vi "Get Json Status.vi"(11 "logger":cluster{"time":string, "message":string}[](array[cluster])) -> (3 "out":string)   [LabVIEW 2019]
uses:
  RT Controls/FPGA State.ctl
  RT Controls/Main Box Config.ctl
  RT Controls/Main Box Status.ctl
  RT Controls/Rotation Status.ctl
  RT Controls/Last Rotation.ctl
  RT Controls/Homing State.ctl
panel:
  out "mainHostAddr":string
  out "logs":cluster{"time":string[], "messages":string[]}
  out "messages":string[](array[string])
  out "time":string[](array[string])
  out "AZEncCounts":u64
  out "watchdogTime":bool
  out "shutdown":bool
  out "current time":timestamp
  out "antWifi":bool
  out "hostComms":bool
  out "buttons":T1
  out "config":T2
  out "errors":T3
  out "time":string
  out "AZPosError":dbl
  out "AZPosReq":dbl
  out "homed":bool
  out "homing":bool
  out "cmd":i8
  out "homeSensor":bool
  out "envSensor":bool
  out "AZEncStatus":u16
  out "subMode":u8
  out "mode":string
  out "modeReq":string
  out "AZLastRot":string
  out "AZPos":dbl
  out "AZEncCounts":u64
  out "autoShutEn":bool
  out "watchdogTim":i32
  out "topBoxComms":bool
  out "hostTimeout":bool
  out "topBoxTimeout":bool
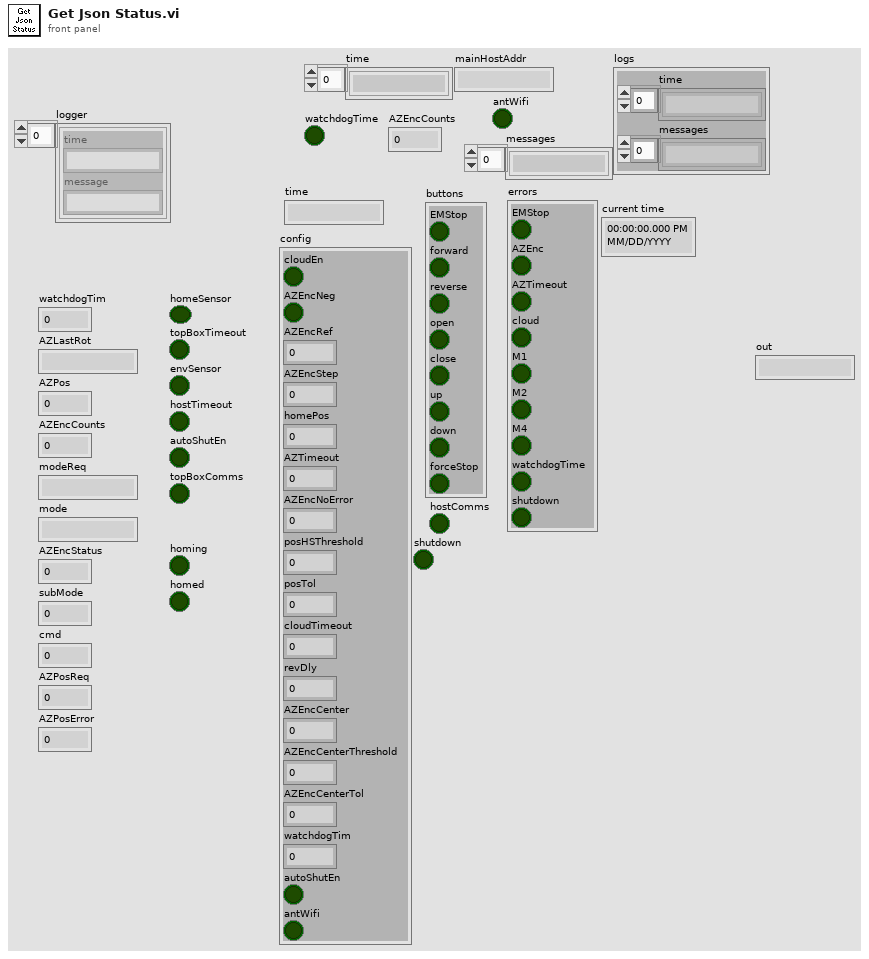
[diagram p1: front panel]
types:
  T1 = cluster{"EMStop":bool, "forward":bool, "reverse":bool, "open":bool, "close":bool, "up":bool, "down":bool, "forceStop":bool}
  T2 = cluster{"cloudEn":bool, "AZEncNeg":bool, "AZEncRef":u64, "AZEncStep":u64, "homePos":dbl, "AZTimeout":u32, "AZEncNoError":u16, "posHSThreshold":dbl, "posTol":dbl, "cloudTimeout":u32, "revDly":u32, "AZEncCenter":u64, "AZEncCenterThreshold":u64, "AZEncCenterTol":u64, "watchdogTim":i32, "autoShutEn":bool, "antWifi":bool}
  T3 = cluster{"EMStop":bool, "AZEnc":bool, "AZTimeout":bool, "cloud":bool, "M1":bool, "M2":bool, "M4":bool, "watchdogTime":bool, "shutdown":bool}
  T4 = typedef "Main Box Status.ctl" = cluster{"RotStatus":T5, "EMButton":bool, "TopComms":bool, "CurAZ":dbl, "At Home":bool, "LastRot":T6, "Cloud":bool, "CurAZEnc":u64, "LastAZ":dbl, "AutoShut":bool, "WDTime":bool, "HomeState":T7}
  T5 = typedef "Rotation Status.ctl" = enum16{"Stop", "Left", "Right", "Homing"}
  T6 = typedef "Last Rotation.ctl" = enum16{"--", "RR", "RL"}
  T7 = typedef "Homing State.ctl" = enum16{"Idle", "SlewFwd", "SlewRev", "SeekFwd", "SeekRev", "AtHome", "FwdWait", "RevWait"}
  T8 = typedef "Main Box Config.ctl" = cluster{"WatchdogTim":i32, "DirRevDel":i32, "Coast":dbl, "HSThres":dbl, "EncCounts360":u64, "HomePos":dbl, "EncRefDeg":dbl, "EncRefCounts":u64, "Tol":dbl, "CloudEn":bool, "AutoShutEn":bool, "RainTim":i32, "AZTimeout":i32, "AZEncPol":enum16{"Positive", "Negative"}}
  T9 = typedef "FPGA State.ctl" = cluster{"mode request":enum16{"stop", "home", "position", "center"}, "az last rotation":enum16{"none", "forward", "reverse"}, "emergency stop":bool, "error?":bool, "errors":cluster{"emergency stop":bool, "encoder":bool, "az timeout":bool, "m1":bool, "m2":bool, "m4":bool}, "az enc counts":u64, "az pos":fxp<+/-,32,2>, "mode":u8, "sub mode":u8, "enc status":u16, "buttons":cluster{"em-stop":bool, "forward":bool, "reverse":bool, "open":bool, "close":bool, "up":bool, "down":bool, "force stop":bool}, "cloud?":bool, "cloud to counter":u32, "az to counter":u32, "env sensor":bool, "home sensor":bool, "rev dly counter":u32, "cmd request":i8, "cmd":i8, "config":cluster{"io.cloud-enable":bool, "io.encoder-negate":bool, "io.encoder-ref":u64, "io.encoder-step":u64, "io.home-pos":fxp<+/-,32,2>, "sm.az-timeout (ms)":u32, "sm.encoder-no-error":u16, "sm.main-pos-hs-thres":fxp<+/-,32,2>, "sm.main-pos-tol":fxp<+/-,32,2>, "sm.cloud-timeout (ms)":u32, "sm.rev-dly (ms)":u32, "io.encoder-center":u64, "sm-main-center-hs-thres":u64, "sm-main-center-tol":u64}, "homing?":bool, "homed?":bool, "az pos req":fxp<+/-,32,2>, "homing wait counter":u32, "config out":cluster{"io.cloud-enable":bool, "io.encoder-negate":bool, "io.encoder-ref":u64, "io.encoder-step":u64, "io.home-pos":fxp<+/-,32,2>, "sm.az-timeout (ms)":u32, "sm.encoder-no-error":u16, "sm.main-pos-hs-thres":fxp<+/-,32,2>, "sm.main-pos-tol":fxp<+/-,32,2>, "sm.cloud-timeout (ms)":u32, "sm.rev-dly (ms)":u32, "io.encoder-center":u64, "sm-main-center-hs-thres":u64, "sm-main-center-tol":u64}, "Chassis Temperature":i16}
  T10 = cluster{"emergency stop":bool, "encoder":bool, "az timeout":bool, "m1":bool, "m2":bool, "m4":bool}
  T11 = cluster{"io.cloud-enable":bool, "io.encoder-negate":bool, "io.encoder-ref":u64, "io.encoder-step":u64, "io.home-pos":fxp<+/-,32,2>, "sm.az-timeout (ms)":u32, "sm.encoder-no-error":u16, "sm.main-pos-hs-thres":fxp<+/-,32,2>, "sm.main-pos-tol":fxp<+/-,32,2>, "sm.cloud-timeout (ms)":u32, "sm.rev-dly (ms)":u32, "io.encoder-center":u64, "sm-main-center-hs-thres":u64, "sm-main-center-tol":u64}
  T12 = cluster{"em-stop":bool, "forward":bool, "reverse":bool, "open":bool, "close":bool, "up":bool, "down":bool, "force stop":bool}
  T13 = cluster{"time":string, "hostComms":bool, "topBoxComms":bool, "mainHostAddr":string, "AZPos":dbl, "AZPosReq":dbl, "AZPosError":dbl, "AZEncCounts":u64, "AZEncStatus":u16, "AZLastRot":string, "mode":string, "modeReq":string, "subMode":u8, "cmd":i8, "buttons":cluster{"EMStop":bool, "forward":bool, "reverse":bool, "open":bool, "close":bool, "up":bool, "down":bool, "forceStop":bool}, "envSensor":bool, "homed":bool, "homing":bool, "homeSensor":bool, "config":cluster{"cloudEn":bool, "AZEncNeg":bool, "AZEncRef":u64, "AZEncStep":u64, "homePos":dbl, "AZTimeout":u32, "AZEncNoError":u16, "posHSThreshold":dbl, "posTol":dbl, "cloudTimeout":u32, "revDly":u32, "AZEncCenter":u64, "AZEncCenterThreshold":u64, "AZEncCenterTol":u64, "watchdogTim":i32, "autoShutEn":bool, "antWifi":bool}, "errors":cluster{"EMStop":bool, "AZEnc":bool, "AZTimeout":bool, "cloud":bool, "M1":bool, "M2":bool, "M4":bool, "watchdogTime":bool, "shutdown":bool}, "logs":cluster{"time":string[], "messages":string[]}}
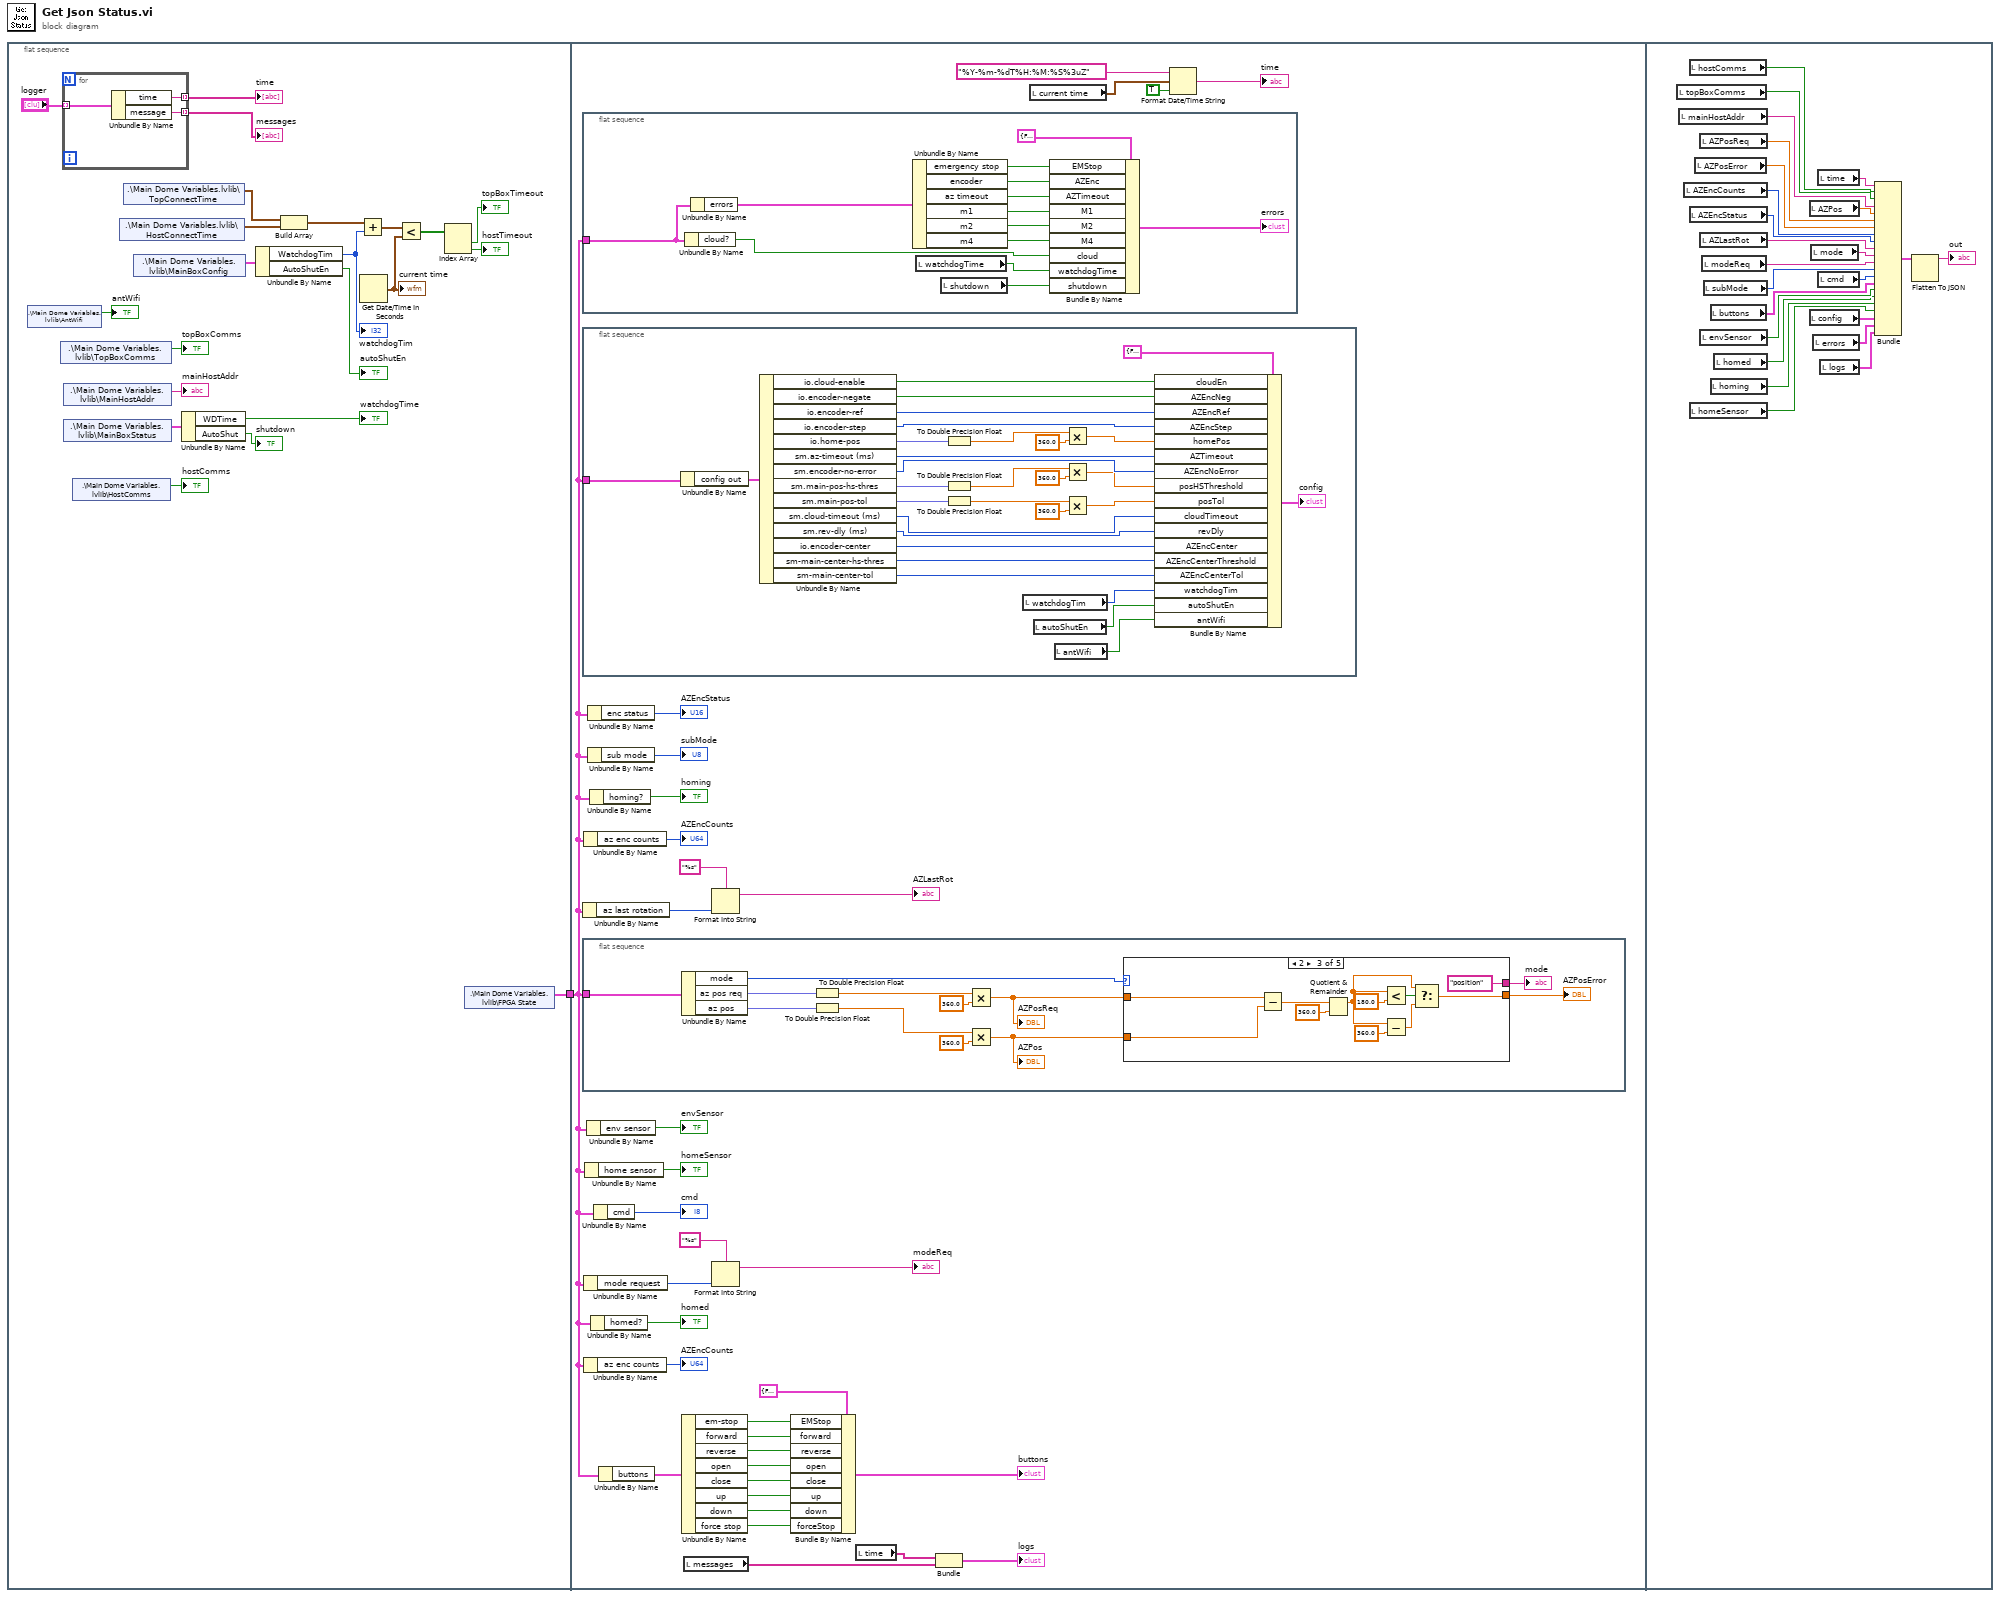
[diagram p0: block diagram]
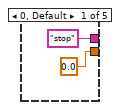
[diagram p2: hidden frame]
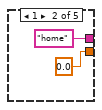
[diagram p3: hidden frame]
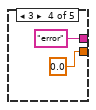
[diagram p4: hidden frame]
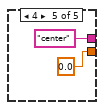
[diagram p5: hidden frame]
diagram:
  n1 = flat-sequence {
    tunnel: [w12] -> w1
    tunnel: w1 -> [w31]
    frame #0 {
      n2 = shared-variable ".\\Main Dome Variables.lvlib\\AntWifi"() -> (→"antWifi":bool)  [unwired: 1 in, 1 out]
      n3 = shared-variable ".\\Main Dome Variables.lvlib\\TopBoxComms"() -> (→"topBoxComms":bool)  [unwired: 1 in, 1 out]
      n4 = for {
        tunnel: "logger" -> [w26] mode=indexing
        tunnel: [w25] -> w4 mode=indexing
        tunnel: [w24] -> w3 mode=indexing
        n5 = Unbundle By Name(w26) -> ("time"=w25:string, "message"=w24:string)
      }
      "time" <- w4
      "messages" <- w3
      n6 = shared-variable ".\\Main Dome Variables.lvlib\\MainHostAddr"() -> (→"mainHostAddr":string)  [unwired: 1 in, 1 out]
      n7 = shared-variable ".\\Main Dome Variables.lvlib\\MainBoxStatus"() -> (w8:T4)  [unwired: 1 in, 1 out]
      n8 = shared-variable ".\\Main Dome Variables.lvlib\\HostComms"() -> (→"hostComms":bool)  [unwired: 1 in, 1 out]
      n9 = shared-variable ".\\Main Dome Variables.lvlib\\HostConnectTime"() -> (w19:timestamp)  [unwired: 1 in, 1 out]
      n10 = shared-variable ".\\Main Dome Variables.lvlib\\TopConnectTime"() -> (w20:timestamp)  [unwired: 1 in, 1 out]
      n11 = shared-variable ".\\Main Dome Variables.lvlib\\MainBoxConfig"() -> (w18:T8)  [unwired: 1 in, 1 out]
      n12 = Unbundle By Name(w8) -> ("WDTime"=→"watchdogTime":bool, "AutoShut"=→"shutdown":bool)
      n13 = Unbundle By Name(w18) -> ("WatchdogTim"=w22:i32, "AutoShutEn"=→"autoShutEn":bool)
      "watchdogTim" <- w22
      n14 = Build Array(w20, w19) -> (w21:timestamp[])
      n15 = Add(x=w21, y=w22) -> (x+y=w23:timestamp[])
      n16 = Get Date/Time In Seconds() -> (seconds since 1Jan1904=w11:timestamp)
      "current time" <- w11
      n17 = Less?(x=w23, y=w11) -> (x < y?=w17:bool[])
      n18 = Index Array(array=w17) -> (element #1=→"topBoxTimeout":bool, element #2=→"hostTimeout":bool)  [unwired: 2 in]
      n19 = shared-variable ".\\Main Dome Variables.lvlib\\FPGA State"() -> (w12:T9)  [unwired: 1 in, 1 out]
    }
    frame #1 {
      n20 = flat-sequence {
        tunnel: w31 -> [w126]
        frame #0 {
          n21 = Unbundle By Name(w126) -> ("cloud?"=w125:bool)
          n22 = Unbundle By Name(w126) -> ("errors"=w134:T10)
          n23 = Unbundle By Name(w134) -> ("emergency stop"=w132:bool, "encoder"=w131:bool, "az timeout"=w130:bool, "m1"=w129:bool, "m2"=w128:bool, "m4"=w127:bool)
          n24 = local read "watchdogTime"() -> (w122:bool)
          n25 = local read "shutdown"() -> (w123:bool)
          n26 = Bundle By Name(cluster=T3 {"EMStop"=FALSE, "AZEnc"=FALSE, "AZTimeout"=FALSE, "cloud"=FALSE, "M1"=FALSE, "M2"=FALSE, "M4"=FALSE, "watchdogTime"=FALSE, "shutdown"=FALSE} ("errors"), "EMStop"=w132, "AZEnc"=w131, "AZTimeout"=w130, "M1"=w129, "M2"=w128, "M4"=w127, "cloud"=w125, "watchdogTime"=w122, "shutdown"=w123) -> (→"errors":T3)
        }
      }
      n27 = flat-sequence {
        tunnel: w31 -> [w95]
        frame #0 {
          n28 = Unbundle By Name(w95) -> ("config out"=w121:T11)
          n29 = Unbundle By Name(w121) -> ("io.cloud-enable"=w119:bool, "io.encoder-negate"=w118:bool, "io.encoder-ref"=w117:u64, "io.encoder-step"=w116:u64, "io.home-pos"=w105:fxp<+/-,32,2>, "sm.az-timeout (ms)"=w115:u32, "sm.encoder-no-error"=w114:u16, "sm.main-pos-hs-thres"=w103:fxp<+/-,32,2>, "sm.main-pos-tol"=w101:fxp<+/-,32,2>, "sm.cloud-timeout (ms)"=w113:u32, "sm.rev-dly (ms)"=w112:u32, "io.encoder-center"=w111:u64, "sm-main-center-hs-thres"=w110:u64, "sm-main-center-tol"=w109:u64)
          n30 = To Double Precision Float(number=w105) -> (double precision float=w98:dbl)
          n31 = To Double Precision Float(number=w103) -> (double precision float=w97:dbl)
          n32 = To Double Precision Float(number=w101) -> (double precision float=w96:dbl)
          n33 = local read "watchdogTim"() -> (w108:i32)
          n34 = local read "autoShutEn"() -> (w94:bool)
          n35 = local read "antWifi"() -> (w92:bool)
          n36 = Multiply(x=w98, y=360.0) -> (x*y=w106:dbl)
          n37 = Multiply(x=w97, y=360.0) -> (x*y=w100:dbl)
          n38 = Multiply(x=w96, y=360.0) -> (x*y=w99:dbl)
          n39 = Bundle By Name(cluster=T2 {"cloudEn"=FALSE, "AZEncNeg"=FALSE, "AZEncRef"=0, "AZEncStep"=0, "homePos"=0.0, "AZTimeout"=0, "AZEncNoError"=0, "posHSThreshold"=0.0, "posTol"=0.0, "cloudTimeout"=0, "revDly"=0, "AZEncCenter"=0, "AZEncCenterThreshold"=0, "AZEncCenterTol"=0, "watchdogTim"=0, "autoShutEn"=FALSE, "antWifi"=FALSE} ("config out"), "cloudEn"=w119, "AZEncNeg"=w118, "AZEncRef"=w117, "AZEncStep"=w116, "homePos"=w106, "AZTimeout"=w115, "AZEncNoError"=w114, "posHSThreshold"=w100, "posTol"=w99, "cloudTimeout"=w113, "revDly"=w112, "AZEncCenter"=w111, "AZEncCenterThreshold"=w110, "AZEncCenterTol"=w109, "watchdogTim"=w108, "autoShutEn"=w94, "antWifi"=w92) -> (→"config":T2)
        }
      }
      n40 = Unbundle By Name(w31) -> ("az last rotation"=w55:enum16{"none", "forward", "reverse"})
      n41 = flat-sequence {
        tunnel: w31 -> [w69]
        frame #0 {
          n42 = Unbundle By Name(w69) -> ("mode"=w67:u8, "az pos req"=w68:fxp<+/-,32,2>, "az pos"=w70:fxp<+/-,32,2>)
          n43 = To Double Precision Float(number=w68) -> (double precision float=w63:dbl)
          n44 = To Double Precision Float(number=w70) -> (double precision float=w72:dbl)
          n45 = Multiply(x=w63, y=360.0 ("number")) -> (x*y=w61:dbl)
          "AZPosReq" <- w61
          n46 = Multiply(x=w72, y=360.0) -> (x*y=w62:dbl)
          "AZPos" <- w62
          n47 = case shown="2" w67 {
            tunnel: ["stop" "home" "position" "error" "center"] -> w65
            tunnel: [0.0 0.0 w80 0.0 0.0] -> w66
            tunnel: w62 -> [_ _ w86 _ _]
            tunnel: w61 -> [_ _ w85 _ _]
            frame 0, Default {
            }
            frame 1 {
            }
            frame 2 {
              n48 = Subtract(x=w85, y=w86) -> (x-y=w83:dbl)
              n49 = Quotient & Remainder(x=w83, y=360.0) -> (x-y*floor(x/y)=w79:dbl)  [unwired: 1 out]
              n50 = Less?(x=w79, y=180.0) -> (x < y?=w81:bool)
              n51 = Subtract(x=w79, y=360.0) -> (x-y=w78:dbl)
              n52 = Select(t=w79, s=w81, f=w78) -> (s? t:f=w80:dbl)
            }
            frame 3 {
            }
            frame 4 {
            }
          }
          "AZPosError" <- w66
          "mode" <- w65
        }
      }
      n53 = Unbundle By Name(w31) -> ("az enc counts"=→"AZEncCounts":u64)
      n54 = Unbundle By Name(w31) -> ("mode request"=w56:enum16{"stop", "home", "position", "center"})
      n55 = Unbundle By Name(w31) -> ("az enc counts"=→"AZEncCounts":u64)
      n56 = Unbundle By Name(w31) -> ("home sensor"=→"homeSensor":bool)
      n57 = Unbundle By Name(w31) -> ("env sensor"=→"envSensor":bool)
      n58 = Unbundle By Name(w31) -> ("enc status"=→"AZEncStatus":u16)
      n59 = Unbundle By Name(w31) -> ("sub mode"=→"subMode":u8)
      n60 = Unbundle By Name(w31) -> ("homing?"=→"homing":bool)
      n61 = Unbundle By Name(w31) -> ("homed?"=→"homed":bool)
      n62 = Unbundle By Name(w31) -> ("cmd"=→"cmd":i8)
      n63 = Unbundle By Name(w31) -> ("buttons"=w45:T12)
      n64 = Unbundle By Name(w45) -> ("em-stop"=w44:bool, "forward"=w43:bool, "reverse"=w42:bool, "open"=w41:bool, "close"=w40:bool, "up"=w39:bool, "down"=w38:bool, "force stop"=w37:bool)
      n65 = local read "messages"() -> (w29:string[])
      n66 = Format Into String(format string="%s", w55) -> (resulting string=→"AZLastRot":string)  [unwired: 2 in, 1 out]
      n67 = Format Into String(format string="%s", w56) -> (resulting string=→"modeReq":string)  [unwired: 2 in, 1 out]
      n68 = Bundle By Name(cluster=T1 {"EMStop"=FALSE, "forward"=FALSE, "reverse"=FALSE, "open"=FALSE, "close"=FALSE, "up"=FALSE, "down"=FALSE, "forceStop"=FALSE} ("buttons"), "EMStop"=w44, "forward"=w43, "reverse"=w42, "open"=w41, "close"=w40, "up"=w39, "down"=w38, "forceStop"=w37) -> (→"buttons":T1)
      n69 = local read "time"() -> (w28:string[])
      n70 = Bundle("time"=w28, "messages"=w29) -> (→"logs":cluster{"time":string[], "messages":string[]})  [unwired: 1 in]
      n71 = local read "current time"() -> (w32:timestamp)
      n72 = Format Date/Time String(time format string (%c)="%Y-%m-%dT%H:%M:%S%3uZ", seconds (now)=w32, UTC format=TRUE) -> (date/time string=→"time":string)
    }
    frame #2 {
      n73 = local read "topBoxComms"() -> (w139:bool)
      n74 = local read "mainHostAddr"() -> (w135:string)
      n75 = local read "AZEncCounts"() -> (w137:u64)
      n76 = local read "hostComms"() -> (w138:bool)
      n77 = local read "AZEncStatus"() -> (w155:u16)
      n78 = local read "homeSensor"() -> (w146:bool)
      n79 = local read "AZPosError"() -> (w156:dbl)
      n80 = local read "AZPosReq"() -> (w157:dbl)
      n81 = local read "AZLastRot"() -> (w154:string)
      n82 = local read "envSensor"() -> (w149:bool)
      n83 = local read "modeReq"() -> (w152:string)
      n84 = local read "subMode"() -> (w151:u8)
      n85 = local read "buttons"() -> (w140:T1)
      n86 = local read "homing"() -> (w147:bool)
      n87 = local read "homed"() -> (w148:bool)
      n88 = local read "AZPos"() -> (w158:dbl)
      n89 = local read "config"() -> (w145:T2)
      n90 = local read "mode"() -> (w153:string)
      n91 = local read "errors"() -> (w144:T3)
      n92 = local read "time"() -> (w141:string)
      n93 = local read "cmd"() -> (w150:i8)
      n94 = local read "logs"() -> (w136:cluster{"time":string[], "messages":string[]})
      n95 = Bundle("time"=w141, "hostComms"=w138, "topBoxComms"=w139, "mainHostAddr"=w135, "AZPos"=w158, "AZPosReq"=w157, "AZPosError"=w156, "AZEncCounts"=w137, "AZEncStatus"=w155, "AZLastRot"=w154, "mode"=w153, "modeReq"=w152, "subMode"=w151, "cmd"=w150, "buttons"=w140, "envSensor"=w149, "homed"=w148, "homing"=w147, "homeSensor"=w146, "config"=w145, "errors"=w144, "logs"=w136) -> (w143:T13)  [unwired: 1 in]
      n96 = Flatten To JSON(anything=w143) -> (JSON string=→"out":string)  [unwired: 2 in, 1 out]
    }
  }
